vi "Parse.vi"(8 "error in (no error)":errorcluster, 10 "Data String":string, 11 "General Parser in":refnum<class "General Parser.lvclass">) -> (0 "error out":errorcluster, 2 "Data Values":dbl[](array[numeric]), 3 "General Parser out":refnum<class "General Parser.lvclass">)   [LabVIEW 2024, in "General Parser.lvclass"]
doc: "General Parser.lvclass:Parse.vi\n\nThis VI takes a string read from an instrument as input and returns an array of channel values.\n\nInstrument Communication Module Version 1.0\nSeptember, 2017 Original Code Consulting David Thomson\n www.originalcode.com"
uses:
  General Parser.lvclass
  General Parser.lvclass/General Parser.ctl
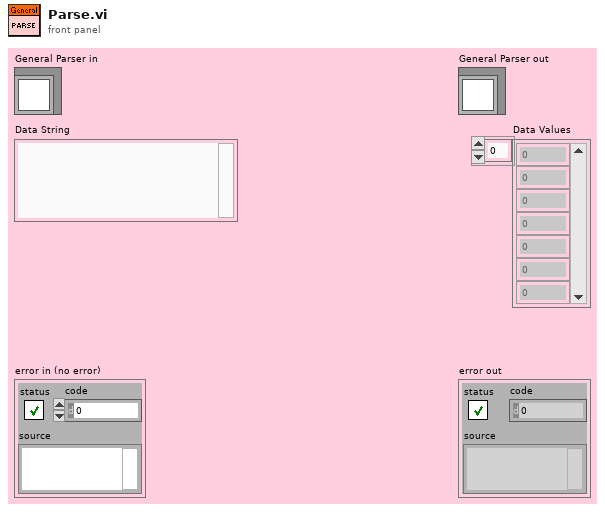
[diagram p1: front panel]
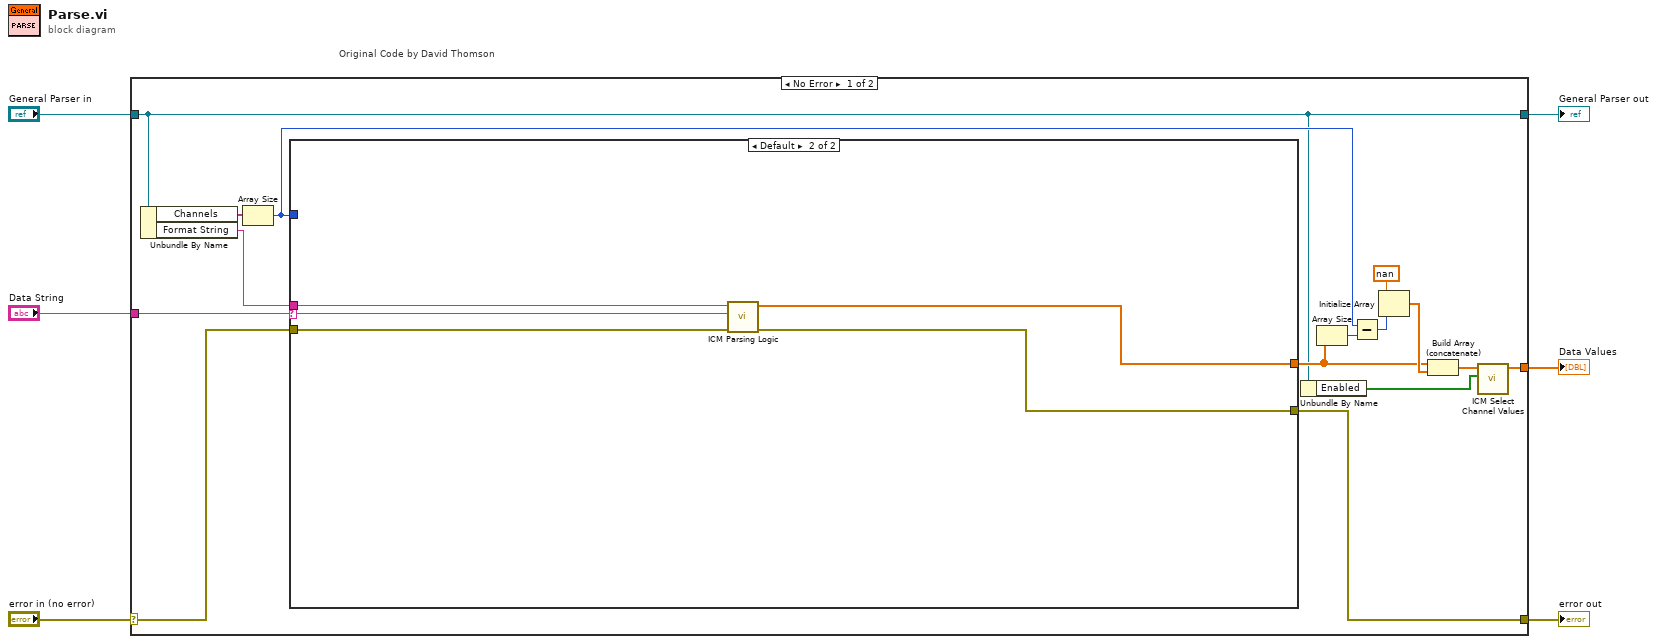
[diagram p0: block diagram]
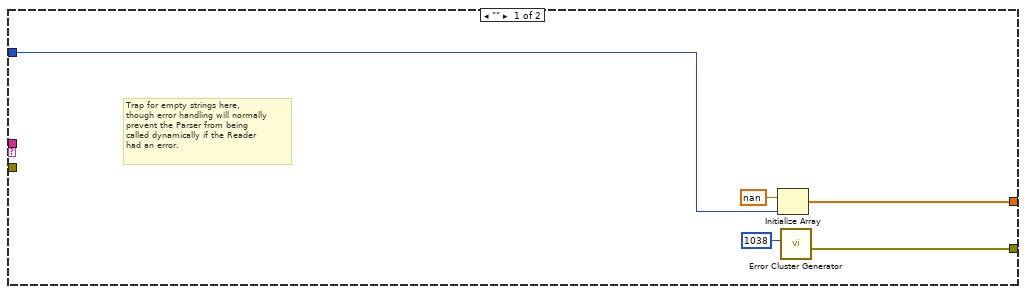
[diagram p2: hidden frame]
diagram:
  n1 = case "Original Code by David Thomson" shown="No Error" "error in (no error)" {
    selector: "error in (no error)" -> [w16 w33]
    tunnel: [w15 w33] -> w5
    tunnel: [w9 w32] -> w3
    tunnel: "General Parser in" -> [w9 w32]
    tunnel: "Data String" -> [w14 _]
    tunnel: [w10 _] -> w1
    frame No Error {
      n2 = Unbundle By Name(w9) -> ("Channels"=w13:string[], "Format String"=w7:string)
      n3 = Array Size(array=w13) -> (size(s)=w12:i32)
      n4 = case shown="Default" w14 {
        selector: w14 -> [_ w30]
        tunnel: w16 -> [_ w28]
        tunnel: [w26 w27] -> w15
        tunnel: [w23 w29] -> w17
        tunnel: w12 -> [w22 _]
        tunnel: w7 -> [_ w31]
        frame "" {
          # "Trap for empty strings here,\nthough error handling will normally\nprevent the Parser from being\ncalled dynamically if the Reader\nhad an error."
          n5 = Initialize Array(nan ("y"), w22) -> (w23:dbl[])
          n6 = call "Error Cluster Generator.vi"("code"=1038) -> ("error out"=w26:errorcluster)  [unwired: 5 in, 1 out]
        }
        frame Default {
          n7 = call "ICM Parsing Logic.vi"("error in (no error)"=w28, "Data String"=w30, "Format String"=w31) -> ("error out"=w27:errorcluster, "Data Values"=w29:dbl[])  [unwired: 7 in]
        }
      }
      n8 = Unbundle By Name(w9) -> ("Enabled"=w8:bool[])
      n9 = Array Size(array=w17) -> (size(s)=w20:i32)
      n10 = Subtract(x=w12, y=w20) -> (x-y=w19:i32)
      n11 = Initialize Array(nan ("y"), w19) -> (w18:dbl[])
      n12 = Build Array (concatenate)(w17, w18) -> (w11:dbl[])
      n13 = call "ICM Select Channel Values.vi"("Enabled"=w8, "Channel Values"=w11) -> ("Enabled Values"=w10:dbl[])  [unwired: 9 in]
    }
    frame Error {
    }
  }
  "error out" <- w5
  "General Parser out" <- w3
  "Data Values" <- w1
